vi "Get Plug-Ins.vi"(8 "error in (no error)":errorcluster, 9 "base path":path, 11 "modle":string) -> (0 "error out":errorcluster, 1 "dup path":path, 3 "s? t:f":refnum<class>, 5 "file or folder exists?":bool)   [LabVIEW 2019, in "TestBench.lvlib" / "TestBench.lvclass"]
uses:
  TestBench.lvclass
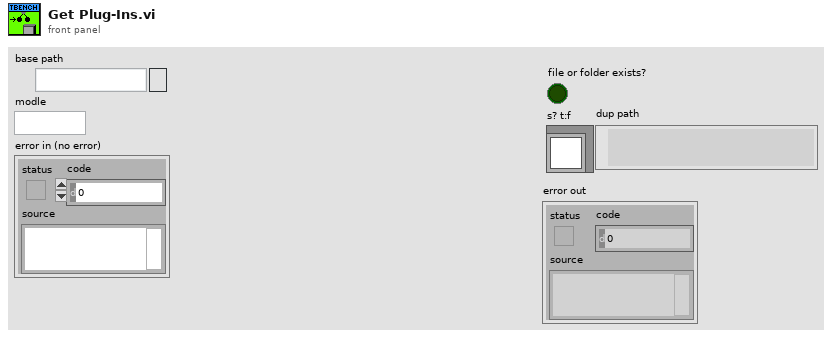
[diagram p1: front panel]
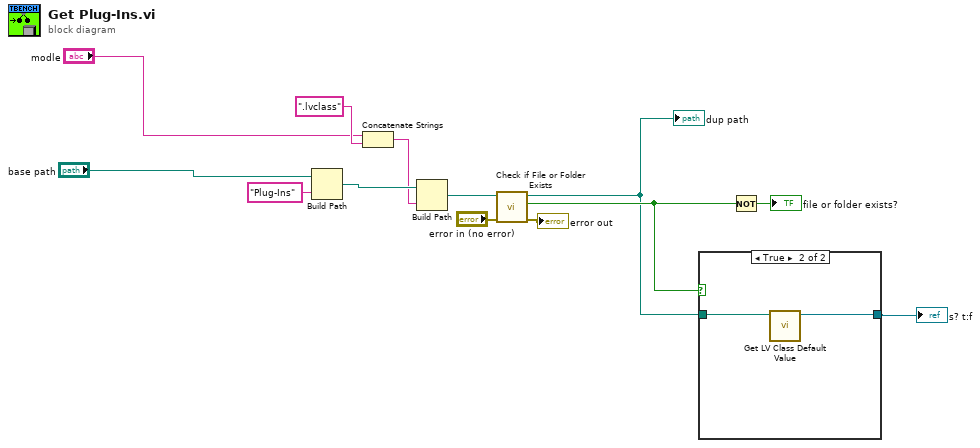
[diagram p0: block diagram]
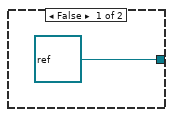
[diagram p2: hidden frame]
diagram:
  n1 = Build Path(base path="base path", name or relative path="Plug-Ins") -> (appended path=w13:path)
  n2 = Concatenate Strings("modle", ".lvclass" ("string")) -> (w12:string)
  n3 = Build Path(base path=w13, name or relative path=w12) -> (appended path=w10:path)
  n4 = call <vilib>:"Check if File or Folder Exists.vi"("error in (no error)"="error in (no error)", "path"=w10) -> ("error out"=→"error out":errorcluster, "file or folder exists?"=w5:bool, "dup path"=w4:path)  [unwired: 7 in]
  "dup path" <- w4
  n5 = case shown="True" w5 {
    tunnel: [refnum<class> refnum ("f") w15] -> w3
    tunnel: w4 -> [_ w16]
    frame False {
    }
    frame True {
      n6 = call <vilib>:"Get LV Class Default Value.vi"("class path"=w16) -> ("object"=w15:refnum<class>)  [unwired: 9 in, 1 out]
    }
  }
  "s? t:f" <- w3
  n7 = Not(x=w5) -> (.not. x?=→"file or folder exists?":bool)
